vi "server_Broadcast.vi"(8 "错误输入（无错误）":errorcluster) -> (0 "error out":errorcluster)   [LabVIEW 2015]
uses:
  Global/SeverGlobal.vi
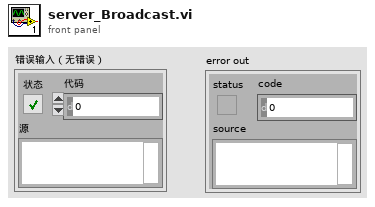
[diagram p1: front panel]
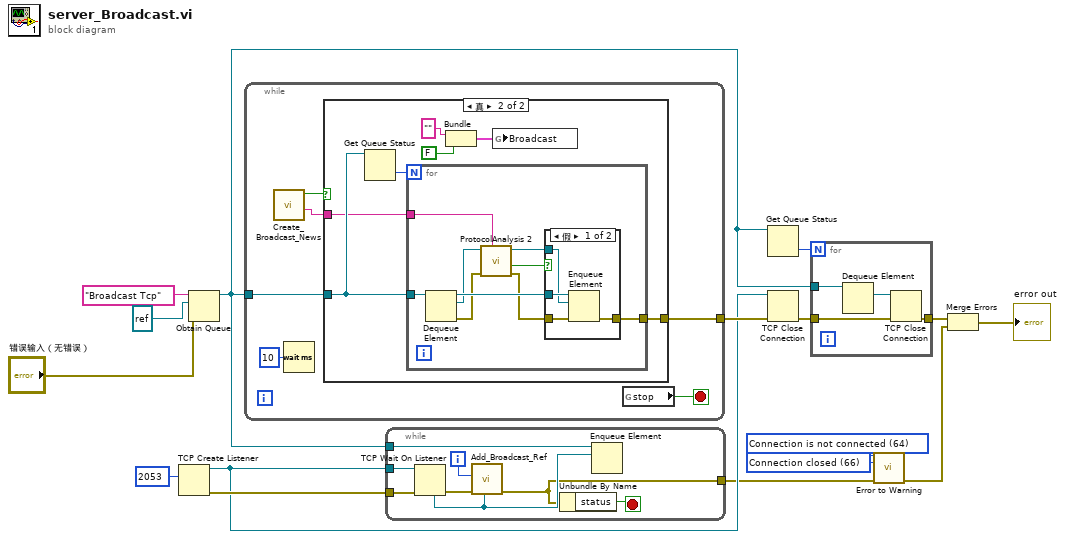
[diagram p0: block diagram]
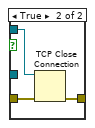
[diagram p3: hidden frame]
diagram:
  w13 = 66 items=["No Error", "Argument Error", "Memory Full", "Out of Zone", "End of File", "File Already Open", "Generic File IO Error", "File Not Found", "File Permission Error", "Disk Full", "Duplicate Path", "Too Many Files Open", "Not Enabled", "Resource File Not Found", "Cannot Add Resource", "Resource Not Found", "Image Not Found", "Image Memory Error", "Pen Does Not Exist", "Config Bad Type", "Config Token Not Found", "Config Parse Error", "Config Memory Error", "Bad External Code Format", "Bad External Code Offset", "External Code Not Present", "Null Window", "Destroy Window Mixup", "Null Menu", "Print Aborted", "Bad Print Record", "Print Driver Error", "Windows Error During Print", "Memory Error During Print", "Print Dialog Error", "Generic Print Error", "Invalid Device Refnum", "Device Not Found", "Device Parameter Error", "Device Unit Error", "Can't Open Device", "Device Call Aborted", "Generic Error", "Cancelled By User", "Object ID Too Low", "Object ID Too High", "Object Not In Heap", "Unknown Heap", "Bad DefProc ID", "DefProc Not In Table", "Message Out Of Range", "Null Method", "Unknown Message", "Manager Call Not Supported", "Bad address", "Connection In progress", "Connection timed out", "Connection is already in progress", "Network attribute not supported", "Network error", "Address in use", "System out of memory", "Connection aborted", "Connection refused", "Connection is not connected", "Connection is already connected", "Connection closed", "Initialize error (interapplication manager)", "Bad occurrence", "Wait on unbound occurrence handler", "Occurrence queue overflow", "Bad path", "Semaphore not signaled", "Unrecognized type (interapplication manager)"] ("2nd Error to Convert")
  w14 = 64 items=["No Error", "Argument Error", "Memory Full", "Out of Zone", "End of File", "File Already Open", "Generic File IO Error", "File Not Found", "File Permission Error", "Disk Full", "Duplicate Path", "Too Many Files Open", "Not Enabled", "Resource File Not Found", "Cannot Add Resource", "Resource Not Found", "Image Not Found", "Image Memory Error", "Pen Does Not Exist", "Config Bad Type", "Config Token Not Found", "Config Parse Error", "Config Memory Error", "Bad External Code Format", "Bad External Code Offset", "External Code Not Present", "Null Window", "Destroy Window Mixup", "Null Menu", "Print Aborted", "Bad Print Record", "Print Driver Error", "Windows Error During Print", "Memory Error During Print", "Print Dialog Error", "Generic Print Error", "Invalid Device Refnum", "Device Not Found", "Device Parameter Error", "Device Unit Error", "Can't Open Device", "Device Call Aborted", "Generic Error", "Cancelled By User", "Object ID Too Low", "Object ID Too High", "Object Not In Heap", "Unknown Heap", "Bad DefProc ID", "DefProc Not In Table", "Message Out Of Range", "Null Method", "Unknown Message", "Manager Call Not Supported", "Bad address", "Connection In progress", "Connection timed out", "Connection is already in progress", "Network attribute not supported", "Network error", "Address in use", "System out of memory", "Connection aborted", "Connection refused", "Connection is not connected", "Connection is already connected", "Connection closed", "Initialize error (interapplication manager)", "Bad occurrence", "Wait on unbound occurrence handler", "Occurrence queue overflow", "Bad path", "Semaphore not signaled", "Unrecognized type (interapplication manager)"] ("1st Error to Convert")
  n1 = TCP Create Listener(10:u32 2053 ("端口")) -> (0:w12:errorcluster, 3:w11:refnum<k5>)  [unwired: 4 in, 1 out]
  n2 = Obtain Queue(name (unnamed)="Broadcast Tcp", element data type=refnum<k5> refnum ("listener ID out"), error in (no error)="错误输入（无错误）") -> (queue out=w2:refnum<queue>)  [unwired: 2 in, 2 out]
  n3 = while {
    tunnel: [w22] -> w15
    tunnel: w2 -> [w21]
    stop <- w19 stop-if-true
    n4 = call "Create_Broadcast_News.vi"() -> ("News"=w17:string, "广播？"=w18:bool)  [unwired: 10 in]
    n5 = Wait (ms)(milliseconds to wait=u32 10 ("等待时间（毫秒）")) -> ()  [unwired: 1 out]
    n6 = case shown="真" w18 {
      tunnel: [_ w29] -> w22
      tunnel: w21 -> [_ w28]
      tunnel: w17 -> [_ w26]
      frame False {
      }
      frame True {
        n7 = Get Queue Status(queue=w28) -> (# elements in queue=w27:i32)  [unwired: 2 in, 7 out]
        n8 = for {
          N: w27 -> [_]
          tunnel: [w36] -> w29
          tunnel: w28 -> [w38]
          tunnel: w26 -> [w30]
          n9 = Dequeue Element(queue=w38) -> (queue out=w37:refnum<queue>, element=w35:refnum<k5>, error out=w34:errorcluster)  [unwired: 2 in, 1 out]
          n10 = call "ProtocolAnalysis 2.vi"("Braodcast_Data"=w30, "error in"=w34, "IP"=w35) -> ("error out"=w32:errorcluster, "Disconnected"=w31:bool, "IP 2"=w33:refnum<k5>)  [unwired: 6 in]
          n11 = case shown="假" w31 {
            tunnel: w37 -> [w42 _]
            tunnel: [w41 w43] -> w36
            tunnel: w33 -> [w40 w45]
            tunnel: w32 -> [w39 w44]
            frame False {
              n12 = Enqueue Element(queue=w42, element=w40, error in (no error)=w39) -> (error out=w41:errorcluster)  [unwired: 1 in, 2 out]
            }
            frame True {
              n13 = TCP Close Connection(connection ID=w45, error in (no error)=w44) -> (error out=w43:errorcluster)  [unwired: 1 in, 1 out]
            }
          }
        }
        n14 = Bundle("", FALSE) -> (w25:cluster{string, bool})  [unwired: 1 in]
        n15 = global write "SeverGlobal.vi" "Broadcast"(w25) -> ()
      }
    }
    n16 = global read "SeverGlobal.vi" "stop"() -> (w19:bool)
  }
  n17 = while {
    tunnel: w11 -> [w53]
    tunnel: w12 -> [w52]
    tunnel: [w47] -> w9
    tunnel: w2 -> [w50]
    i -> [w46]
    stop <- w51 stop-if-true
    n18 = TCP Wait On Listener(8:w52, 11:w53) -> (0:w48:errorcluster, 4:w49:refnum<k5>)  [unwired: 2 in, 3 out]
    n19 = call "Add_Broadcast_Ref.vi"("TCP Ref"=w49, "error in"=w48, "index"=w46) -> ("error out"=w47:errorcluster)  [unwired: 8 in]
    n20 = Unbundle By Name(w47) -> ("status"=w51:bool)
    n21 = Enqueue Element(queue=w50, element=w49) -> ()  [unwired: 2 in, 3 out]
  }
  n22 = Get Queue Status(queue=w2) -> (# elements in queue=w4:i32)  [unwired: 2 in, 7 out]
  n23 = TCP Close Connection(connection ID=w11, error in (no error)=w15) -> (error out=w10:errorcluster)  [unwired: 1 in, 1 out]
  n24 = for {
    N: w4 -> [_]
    tunnel: w10 -> [w57]
    tunnel: [w56] -> w8
    tunnel: w2 -> [w55]
    n25 = Dequeue Element(queue=w55) -> (element=w54:refnum<k5>)  [unwired: 2 in, 3 out]
    n26 = TCP Close Connection(connection ID=w54, error in (no error)=w57) -> (error out=w56:errorcluster)  [unwired: 1 in, 1 out]
  }
  n27 = call <vilib>:"Error to Warning.vi"("1st Error to Convert"=w14, "2nd Error to Convert"=w13, "error in"=w9) -> ("warning out"=w7:errorcluster)  [unwired: 12 in]
  n28 = Merge Errors(w8, w7) -> (→"error out":errorcluster)
